vi "CompleteWavefoem(SubVI).vi"(10 "dt":dbl=0.001, 11 "Array":waveform(dbl)[](array[waveform])) -> (3 "Waveform":waveform(dbl))   [LabVIEW 2021]
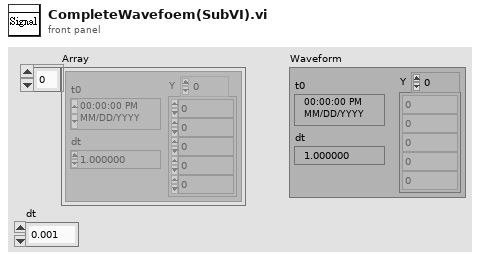
[diagram p1: front panel]
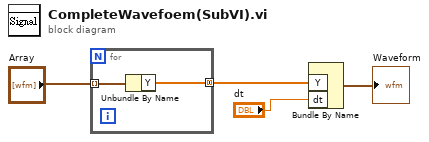
[diagram p0: block diagram]
diagram:
  n1 = for {
    tunnel: [w6] -> w3 mode=concatenating
    tunnel: "Array" -> [w5] mode=indexing
    n2 = Unbundle By Name(w5) -> ("Y"=w6:dbl[])
  }
  n3 = Bundle By Name("Y"=w3, "dt"="dt") -> (→"Waveform":waveform(dbl))  [unwired: 1 in]
